vi "Main.vi"() -> ()   [LabVIEW 2014]
uses:
  Untitled Project 8/Kontrole/StanjeEnc.ctl
panel:
  in  "access (0:read/write)":enum16{"read/write", "read-only", "write-only"}(ring)
  in  "operation (0:open)":T1(ring)
  in  "file path (use dialog)":path
  out "x/y":dbl
  out "Signal":dynamicdata(graph)=[{"t0"=timestamp(0 s since 1904-01-01), "dt"=0.005, "Y"=array[5001 elements], "attributes"=variant("NI_ChannelName"=variant(string "PWM izlaz"))}]
  in  "Stop Button":bool
  in  "Rezolucija":dbl=4000.0
  in  "Precnik":dbl=90.0
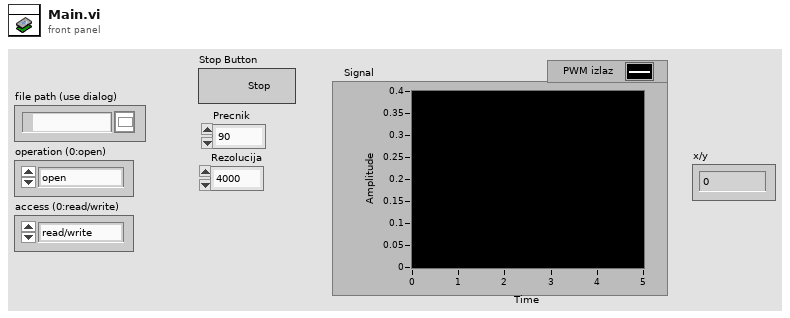
[diagram p1: front panel]
types:
  T1 = enum16{"open", "replace", "create", "open or create", "replace or create", "replace or create with confirmation"}
  T2 = typedef "StanjeEnc.ctl" = enum16{"Inicijalizacija", "Citaj", "Reset"}
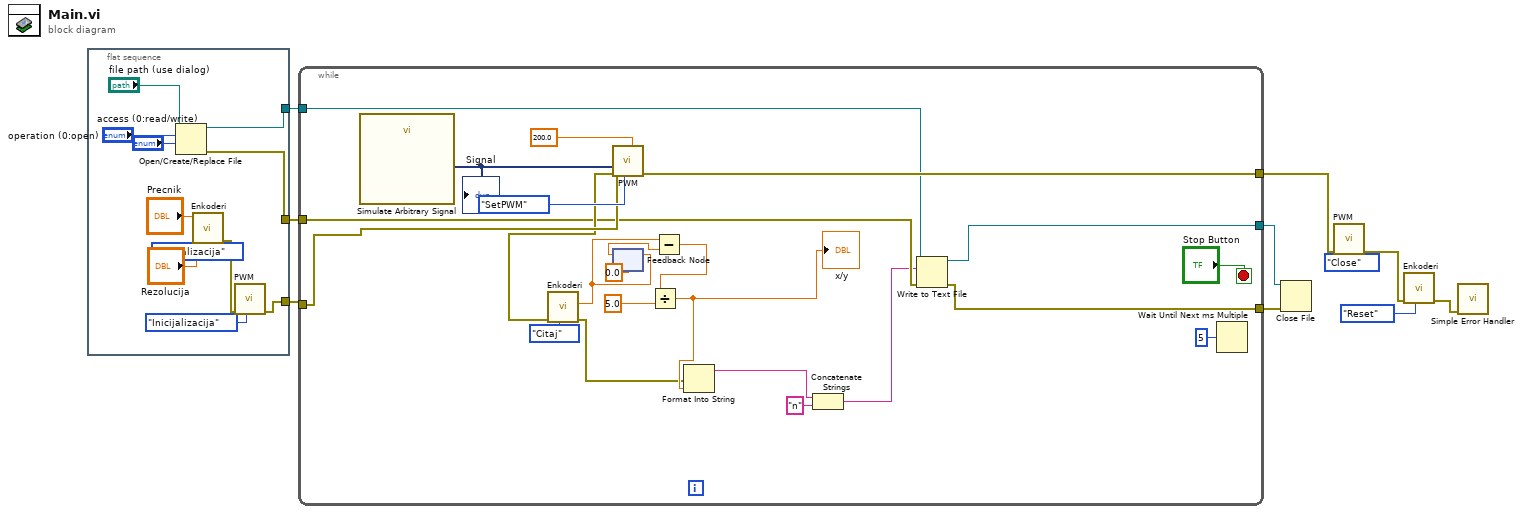
[diagram p0: block diagram]
diagram:
  n1 = flat-sequence {
    tunnel: [w16] -> w10
    tunnel: [w12] -> w4
    tunnel: [w11] -> w3
    frame #0 {
      n2 = Open/Create/Replace File(file path (use dialog)="file path (use dialog)", operation (0:open)="operation (0:open)", access (0:read/write)="access (0:read/write)") -> (refnum out=w11:refnum<file>, error out=w12:errorcluster)  [unwired: 3 in, 1 out]
      n3 = call "Enkoderi.vi"("Enum 2"=StanjeEnc."Inicijalizacija", "Rezolucija"="Rezolucija", "Precnik"="Precnik") -> ("error out 2"=w17:errorcluster)  [unwired: 6 in, 2 out]
      n4 = call "PWM.vi"("Enum"=enum16{"Inicijalizacija", "SetPWM", "Close"}."Inicijalizacija", "error in (no error) 2"=w17) -> ("error out 2"=w16:errorcluster)  [unwired: 9 in]
    }
  }
  n5 = while {
    tunnel: w10 -> [w33]
    tunnel: [w32] -> w5
    tunnel: w4 -> [w30]
    tunnel: w3 -> [w29]
    tunnel: [w27] -> w2
    tunnel: [w26] -> w1
    stop <- "Stop Button" stop-if-true
    n6 = call "Simulate Arbitrary Signal"() -> ("Signal"=w35:dynamicdata)  [unwired: 9 in, 2 out]
    "Signal" <- w35
    n7 = call "PWM.vi"("Frequency [Hz] 2"=200.0, "Enum"=enum16{"Inicijalizacija", "SetPWM", "Close"}."SetPWM", "error in (no error) 2"=w33, "Duty Cycle motor 1"=w35) -> ("error out 2"=w32:errorcluster)  [unwired: 7 in]
    n8 = call "Enkoderi.vi"("Enum 2"=StanjeEnc."Citaj", "error in (no error) 2"=w32) -> ("error out 2"=w25:errorcluster, "Levi Enc"=w34:dbl)  [unwired: 7 in, 1 out]
    n9 = feedback #1(0.0 ("Levi Enc")) -> (w37:dbl)
    n10 = feedback-in #1(w34) -> ()
    n11 = Subtract(x=w34, y=w37) -> (x-y=w36:dbl)
    n12 = Divide(x=w36, y=5.0) -> (x/y=w28:dbl)
    "x/y" <- w28
    n13 = Format Into String(error in=w25, w28) -> (resulting string=w23:string)  [unwired: 2 in, 1 out]
    n14 = Concatenate Strings(w23, "n" ("string")) -> (w22:string)
    n15 = Write to Text File(file (use dialog)=w29, text=w22, error in=w30) -> (refnum out=w26:refnum<file>, error out=w27:errorcluster)  [unwired: 1 in, 1 out]
    n16 = Wait Until Next ms Multiple(millisecond multiple=u32 5) -> ()  [unwired: 1 out]
  }
  n17 = Close File(refnum=w1, error in=w2) -> ()  [unwired: 2 out]
  n18 = call "PWM.vi"("Enum"=enum16{"Inicijalizacija", "SetPWM", "Close"}."Close", "error in (no error) 2"=w5) -> ("error out 2"=w9:errorcluster)  [unwired: 9 in]
  n19 = call "Enkoderi.vi"("Enum 2"=StanjeEnc."Reset", "error in (no error) 2"=w9) -> ("error out 2"=w6:errorcluster)  [unwired: 7 in, 2 out]
  n20 = call <vilib>:"Simple Error Handler.vi"("error in (no error)"=w6) -> ()  [unwired: 4 in, 5 out]
